vi "BRig_dataMTrig_CueLed_N.vi"() -> (2 "output_CueLed_N":i32)   [LabVIEW 2014]
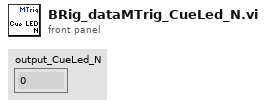
[diagram p1: front panel]
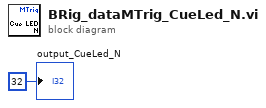
[diagram p0: block diagram]
diagram:
  "output_CueLed_N" <- 32 ("output_iBlock")
